vi "Rotate Drive.vi"(8 "Command Info In":T1, 11 "Degrees":dbl) -> (0 "Command Info Out":T1)   [LabVIEW 2019]
uses:
  <vilib>/Rock Robotics/WPI/Framework/Command Status Info.ctl
  <vilib>/Rock Robotics/WPI/Framework/Completion Status.ctl
  <vilib>/Rock Robotics/WPI/Framework/Completion Notifier.ctl
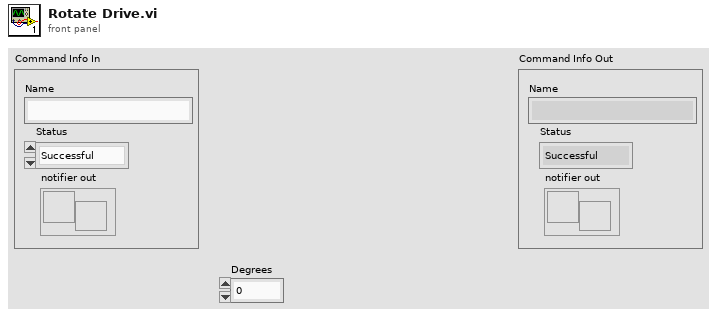
[diagram p1: front panel]
types:
  T1 = typedef "Command Status Info.ctl" = cluster{"Name":string, "Status":T2, "notifier out":T3}
  T2 = typedef "Completion Status.ctl" = enum16{"Successful", "Aborted", "Incomplete"}
  T3 = typedef "Completion Notifier.ctl" = refnum<notifier>
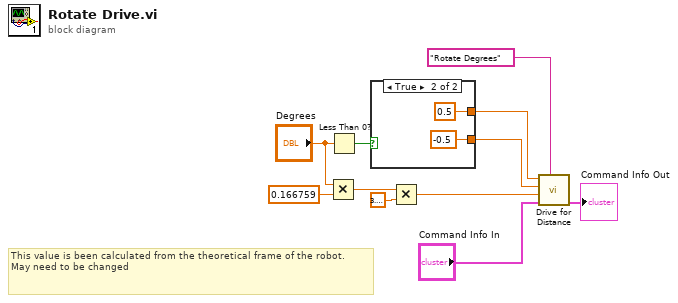
[diagram p0: block diagram]
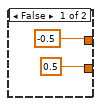
[diagram p2: hidden frame]
diagram:
  # "This value is been calculated from the theoretical frame of the robot.\nMay need to be changed"
  n1 = Multiply(x="Degrees", y=0.166759) -> (x*y=w6:dbl)
  n2 = Less Than 0?(x="Degrees") -> (x < 0?=w1:bool)
  n3 = case shown="True" w1 {
    tunnel: [-0.5 ("Left Setpoint") 0.5 ("Left Setpoint")] -> w11
    tunnel: [0.5 ("Right Setpoint") -0.5 ("Right Setpoint")] -> w10
    frame False {
    }
    frame True {
    }
  }
  n4 = Multiply(x=w6, y=3.141592653589793) -> (x*y=w5:dbl)
  n5 = call "Drive for Distance.vi"("Description"="Rotate Degrees", "Command Info In"="Command Info In", "Distance (inches)"=w5, "Right Setpoint"=w10, "Left Setpoint"=w11) -> ("Command Info Out"=→"Command Info Out":T1)  [unwired: 6 in]
